vi "ATF-CS- Build file folder for datalog.vi"(8 "error in (no error)":errorcluster, 10 "Base Path":path, 11 "File Name":string) -> (0 "error out":errorcluster, 2 "Result File path":path, 3 "Result Folder path":path)   [LabVIEW 2022 SP3]
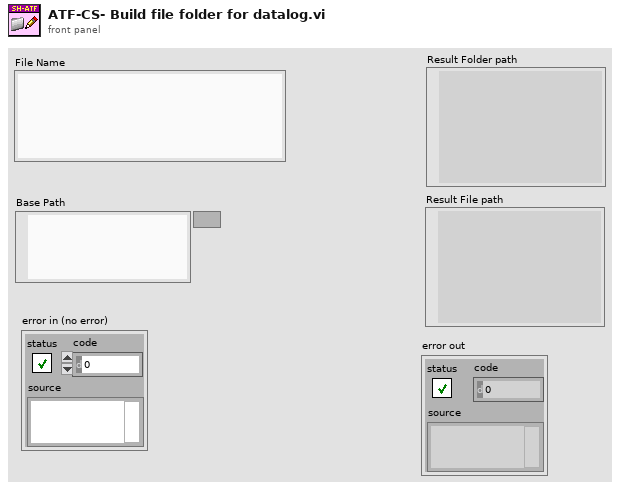
[diagram p1: front panel]
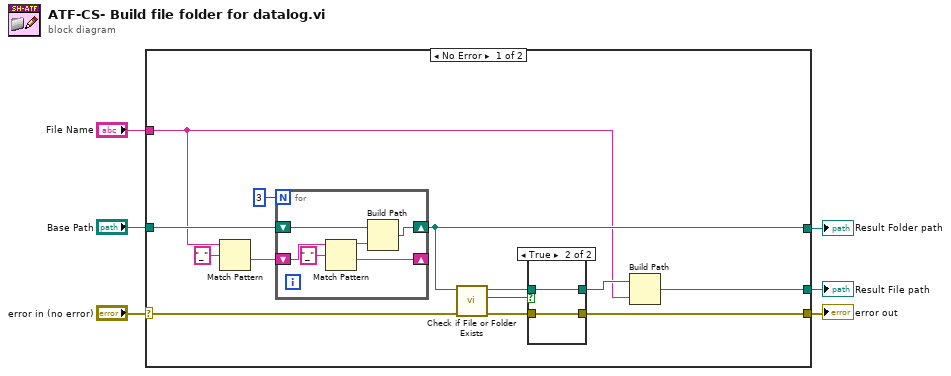
[diagram p0: block diagram]
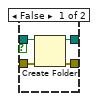
[diagram p2: hidden frame]
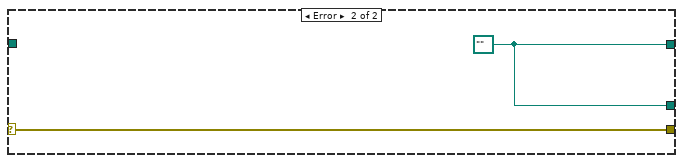
[diagram p3: hidden frame]
diagram:
  n1 = case shown="No Error" "error in (no error)" {
    selector: "error in (no error)" -> [w13 w33]
    tunnel: [w16 w33] -> w5
    tunnel: [w12 w32] -> w4
    tunnel: [w15 w32] -> w3
    tunnel: "File Name" -> [w8 _]
    tunnel: "Base Path" -> [w18 _]
    frame No Error {
      n2 = Match Pattern(string=w8, regular expression="_" ("search string/char (-)")) -> (after substring=w7:string)  [unwired: 1 in, 3 out]
      n3 = for {
        N: 3 -> [_]
        shift-right: [w28] -> _
        shift-left: w7 -> [w26]
        shift-right: [w29] -> w12
        shift-left: w18 -> [w30]
        n4 = Match Pattern(string=w26, regular expression="_" ("search string/char (-)")) -> (before substring=w27:string, after substring=w28:string)  [unwired: 1 in, 2 out]
        n5 = Build Path(base path=w30, name or relative path=w27) -> (appended path=w29:path)
      }
      n6 = call <vilib>:"Check if File or Folder Exists.vi"("error in (no error)"=w13, "path"=w12) -> ("error out"=w10:errorcluster, "file or folder exists?"=w9:bool, "dup path"=w11:path)  [unwired: 7 in]
      n7 = case shown="True" w9 {
        tunnel: [w23 w24] -> w16
        tunnel: [w22 w25] -> w14
        tunnel: w11 -> [w21 w25]
        tunnel: w10 -> [w20 w24]
        frame False {
          n8 = Create Folder(path (use dialog)=w21, error in=w20) -> (created path=w22:path, error out=w23:errorcluster)  [unwired: 1 in, 1 out]
        }
        frame True {
        }
      }
      n9 = Build Path(base path=w14, name or relative path=w8) -> (appended path=w15:path)
    }
    frame Error {
      w32 = path "" ("appended path")
    }
  }
  "error out" <- w5
  "Result Folder path" <- w4
  "Result File path" <- w3
